vi "MessageIn_Communication.vi"(8 "Error In":errorcluster, 10 "Message In":string, 11 "Spaceship in":refnum<class "Spaceship.lvclass">) -> (0 "Error Out":errorcluster, 3 "Spaceship out":refnum<class "Spaceship.lvclass">)   [LabVIEW 2021, in "Spaceship.lvclass"]
doc: "Enqueue string message into class objet queue."
uses:
  Spaceship.lvclass
  Spaceship.lvclass/Spaceship.ctl
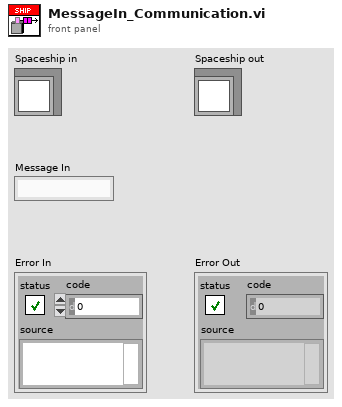
[diagram p1: front panel]
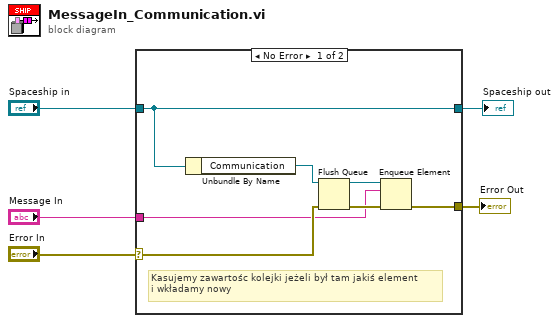
[diagram p0: block diagram]
diagram:
  n1 = case shown="No Error" "Error In" {
    selector: "Error In" -> [w10 w14]
    tunnel: [w7 w14] -> w4
    tunnel: [w12 w13] -> w2
    tunnel: "Spaceship in" -> [w12 w13]
    tunnel: "Message In" -> [w6 _]
    frame No Error {
      # "Kasujemy zawartośc kolejki jeżeli był tam jakiś element \ni wkładamy nowy"
      n2 = Unbundle By Name(w12) -> ("Communication"=w11:refnum<queue>)
      n3 = Flush Queue(queue=w11, error in (no error)=w10) -> (queue out=w8:refnum<queue>, error out=w9:errorcluster)  [unwired: 1 out]
      n4 = Enqueue Element(queue=w8, element=w6, error in (no error)=w9) -> (error out=w7:errorcluster)  [unwired: 1 in, 2 out]
    }
    frame Error {
    }
  }
  "Error Out" <- w4
  "Spaceship out" <- w2
